vi "Logitech F310.vi"(6 "error in (no error)":errorcluster, 8 "refnum name":string) -> (0 "Buttons":T2, 1 "D-Pad Buttons":T1, 2 "D-Pad":cluster{"X":dbl, "Y":dbl}, 3 "Right Stick":cluster{"X":dbl, "Y":dbl}, 4 "error out":errorcluster, 5 "Left Stick":cluster{"X":dbl, "Y":dbl})   [LabVIEW 2012]
uses:
  <vilib>/Rock Robotics/WPI/Joystick/WPI_JoystickGetSetRefNum.vi
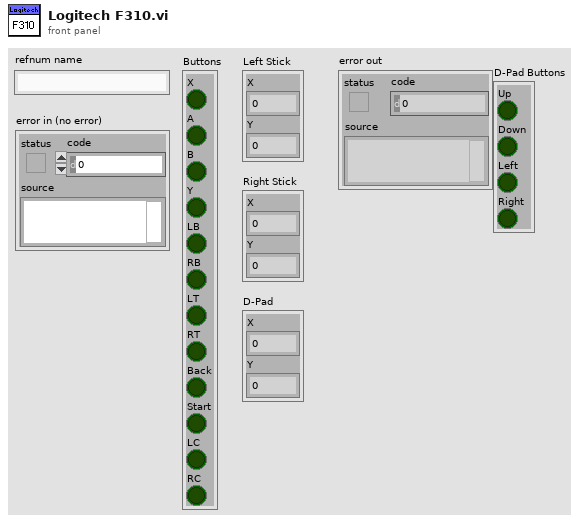
[diagram p1: front panel]
types:
  T1 = cluster{"Up":bool, "Down":bool, "Left":bool, "Right":bool}
  T2 = cluster{"X":bool, "A":bool, "B":bool, "Y":bool, "LB":bool, "RB":bool, "LT":bool, "RT":bool, "Back":bool, "Start":bool, "LC":bool, "RC":bool}
  T3 = typedef "WPI_JoystickDevRef.ctl" = cluster{"Device":T4}
  T4 = typedef "WPI_JoystickDeviceEnum.ctl" = enum16{"USB 1", "USB 2", "USB 3", "USB 4", "Kinect 1", "Kinect 2"}
  T5 = typedef "WPI_JoystickButtonState.ctl" = cluster{"Button 1":bool, "Button 2":bool, "Button 3":bool, "Button 4":bool, "Button 5":bool, "Button 6":bool, "Button 7":bool, "Button 8":bool, "Button 9":bool, "Button 10":bool, "Button 11":bool, "Button 12":bool}
  T6 = cluster{"axis 1 (x)":dbl, "axis 2 (y)":dbl, "axis 3 (throttle)":dbl, "axis 4":dbl, "axis 5":dbl, "axis 6":dbl}
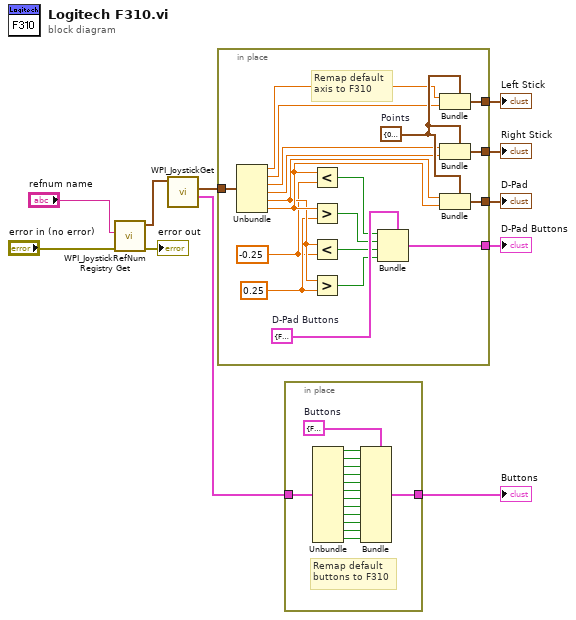
[diagram p0: block diagram]
diagram:
  n1 = call <vilib>:"WPI_JoystickRefNum Registry Get.vi"("error in (no error)"="error in (no error)", "refnum name"="refnum name") -> ("error out"=→"error out":errorcluster, "JoystickDevRef"=w11:T3)  [unwired: 8 in]
  n2 = call <vilib>:"WPI_JoystickGet.vi"("JoystickDevRef"=w11) -> ("Buttons"=w9:T5, "Axes"=w10:T6)  [unwired: 4 in, 1 out]
  n3 = in-place {
    in-place-border: w10 -> [w30]
    in-place-border: [w29] -> w5
    in-place-border: [w28] -> w4
    in-place-border: [w26] -> w3
    in-place-border: [w20] -> w1
    w21 = -0.25 ("y")
    w22 = 0.25 ("y")
    w25 = T1 {"Up"=FALSE, "Down"=FALSE, "Left"=FALSE, "Right"=FALSE}  # D-Pad Buttons
    w27 = cluster{"X":dbl, "Y":dbl} {"X"=0.0, "Y"=0.0}  # Points
    # "Remap default\naxis to F310"
    n4 = Unbundle(w30) -> ("axis 1 (x)"=w15:dbl, "axis 2 (y)"=w14:dbl, "axis 3 (throttle)"=w13:dbl, "axis 4"=w12:dbl, "axis 5"=w23:dbl, "axis 6"=w24:dbl)
    n5 = Less?(x=w24, y=w21) -> (x < y?=w18:bool)
    n6 = Greater?(x=w24, y=w22) -> (0:w19:bool)
    n7 = Less?(x=w23, y=w21) -> (x < y?=w16:bool)
    n8 = Greater?(x=w23, y=w22) -> (0:w17:bool)
    n9 = Bundle(cluster=w25, "Up"=w18, "Down"=w19, "Left"=w16, "Right"=w17) -> (w20:T1)
    n10 = Bundle(cluster=w27, "X"=w15, "Y"=w14) -> (w29:cluster{"X":dbl, "Y":dbl})
    n11 = Bundle(cluster=w27, "X"=w13, "Y"=w12) -> (w28:cluster{"X":dbl, "Y":dbl})
    n12 = Bundle(cluster=w27, "X"=w23, "Y"=w24) -> (w26:cluster{"X":dbl, "Y":dbl})
  }
  "Left Stick" <- w5
  "Right Stick" <- w4
  "D-Pad" <- w3
  "D-Pad Buttons" <- w1
  n13 = in-place {
    in-place-border: w9 -> [w45]
    in-place-border: [w31] -> w2
    w44 = T2 {"X"=FALSE, "A"=FALSE, "B"=FALSE, "Y"=FALSE, "LB"=FALSE, "RB"=FALSE, "LT"=FALSE, "RT"=FALSE, "Back"=FALSE, "Start"=FALSE, "LC"=FALSE, "RC"=FALSE}  # Buttons
    # "Remap default\nbuttons to F310"
    n14 = Unbundle(w45) -> ("Button 1"=w43:bool, "Button 2"=w42:bool, "Button 3"=w41:bool, "Button 4"=w40:bool, "Button 5"=w39:bool, "Button 6"=w38:bool, "Button 7"=w37:bool, "Button 8"=w36:bool, "Button 9"=w35:bool, "Button 10"=w34:bool, "Button 11"=w33:bool, "Button 12"=w32:bool)
    n15 = Bundle(cluster=w44, "X"=w43, "A"=w42, "B"=w41, "Y"=w40, "LB"=w39, "RB"=w38, "LT"=w37, "RT"=w36, "Back"=w35, "Start"=w34, "LC"=w33, "RC"=w32) -> (w31:T2)
  }
  "Buttons" <- w2
